vi "4Pi Obj Lock - Get Cross Correlation.vi"(0 "Ref FFT image":T1, 5 "Cur FFT Image":T1, 7 "FFT CC image":T1, 9 "iFFT image":T1, 11 "error in (no error)":errorcluster, 12 "CC image":T1) -> (4 "Max CC":sgl, 10 "CC image Out":T1, 15 "error out":errorcluster)   [LabVIEW 2021]
uses:
  <vilib>/vision/Image Controls.llb/IMAQ Image.ctl
  <vilib>/vision/NI_Vision_Development_Module.lvlib
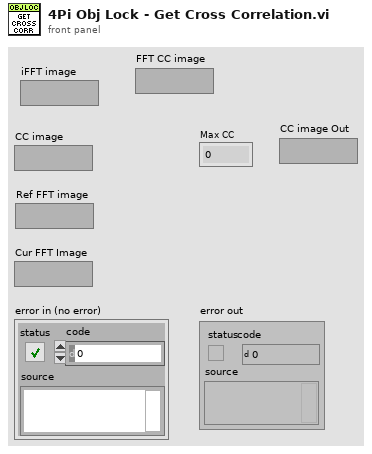
[diagram p1: front panel]
types:
  T1 = typedef "IMAQ Image.ctl" = refnum<image>
  T2 = enum32{"Real", "Imaginary", "Magnitude", "Phase"}
  T3 = cluster{"histogram":u32[], "Minimal Value":sgl, "Maximal Value":sgl, "Starting Value":sgl, "Interval Width":sgl, "Mean Value":sgl, "Standard  Variation":sgl, "Area (pixels)":i32}
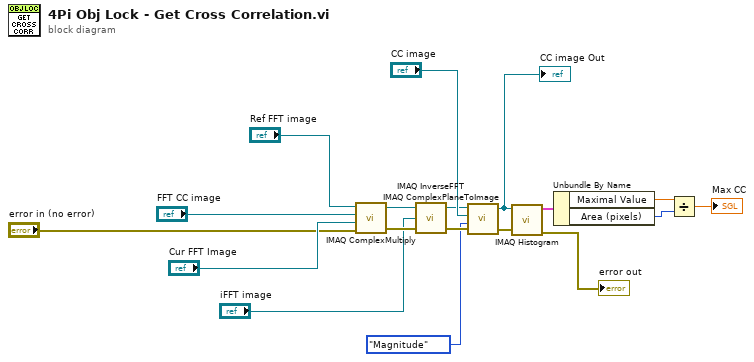
[diagram p0: block diagram]
diagram:
  n1 = call "IMAQ ComplexMultiply"("Image Src A"="Ref FFT image", "Image Dst"="FFT CC image", "Image Src B"="Cur FFT Image", "error in (no error)"="error in (no error)") -> ("Image Dst Out"=w9:T1, "error out"=w14:errorcluster)  [unwired: 3 in]
  n2 = call "IMAQ InverseFFT"("error in (no error)"=w14, "Image Dst"="iFFT image", "Image Src"=w9) -> ("error out"=w15:errorcluster, "Image Dst Out"=w8:T1)  [unwired: 1 in]
  n3 = call "IMAQ ComplexPlaneToImage"("error in (no error)"=w15, "Plane"=T2."Magnitude", "Image Dst"="CC image", "Image Src"=w8) -> ("error out"=w16:errorcluster, "Image Dst Out"=w6:T1)  [unwired: 1 in]
  "CC image Out" <- w6
  n4 = call "IMAQ Histogram"("error in (no error)"=w16, "Image"=w6) -> ("error out"=→"error out":errorcluster, "Histogram Report"=w5:T3)  [unwired: 8 in]
  n5 = Unbundle By Name(w5) -> ("Maximal Value"=w4:sgl, "Area (pixels)"=w3:i32)
  n6 = Divide(x=w4, y=w3) -> (x/y=→"Max CC":sgl)
